vi "Editor Initialize.vi"(0 "Color Ramp Cluster in":T1={"Color Ramp Style"=enum."None", "Color Ramp Array"=[16711934, 393471, 57855, 4390754, 16449346, 16744722, 16711680], "Color Ramp Index"=[45, 91, 133, 175, 219, 255], "Interpolate?"=FALSE, "Logarithm?"=FALSE}, 1 "Fixed Slider Ref":refnum<vi>, 2 "Fixed Color Ref Array":refnum<vi>[](array[refnum]), 3 "Fixed Numeric Ref Array":refnum<vi>[](array[refnum]), 9 "Range In":cluster{"Max":sgl, "Min":sgl}, 11 "error in (no error)":errorcluster, 12 "Slider Ref Array":refnum<vi>[](array[refnum]), 13 "Color Ref Array":refnum<vi>[](array[refnum]), 14 "Numeric Ref Array":refnum<vi>[](array[refnum])) -> (4 "Color Ramp Cluster out":T1={"Color Ramp Style"=enum."None", "Color Ramp Array"=[16711934, 393471, 57855, 4390754, 16449346, 16744722, 16711680], "Color Ramp Index"=[45, 91, 133, 175, 219, 255], "Interpolate?"=FALSE, "Logarithm?"=FALSE}, 10 "Active Slider ID":i32, 15 "error out":errorcluster)   [LabVIEW 2020, in "3D Plot.lvclass"]
uses:
  3D Plot.lvclass
  Color Ramp Cluster.ctl
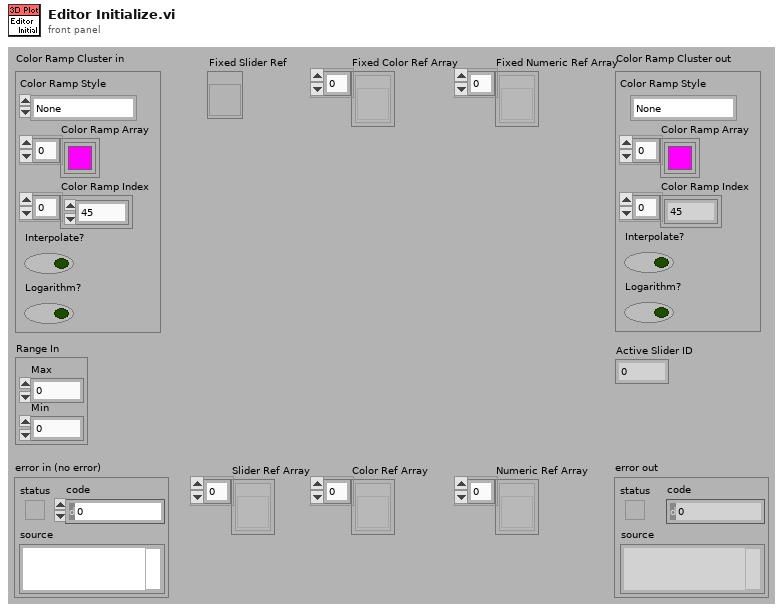
[diagram p1: front panel]
types:
  T1 = typedef "3D Plot.lvclass/Color Ramp Cluster.ctl" = cluster{"Color Ramp Style":enum16{"None", "Shaded", "Color spectrum", "Grey scale", "Custom"}, "Color Ramp Array":u32[], "Color Ramp Index":i32[], "Interpolate?":bool, "Logarithm?":bool}
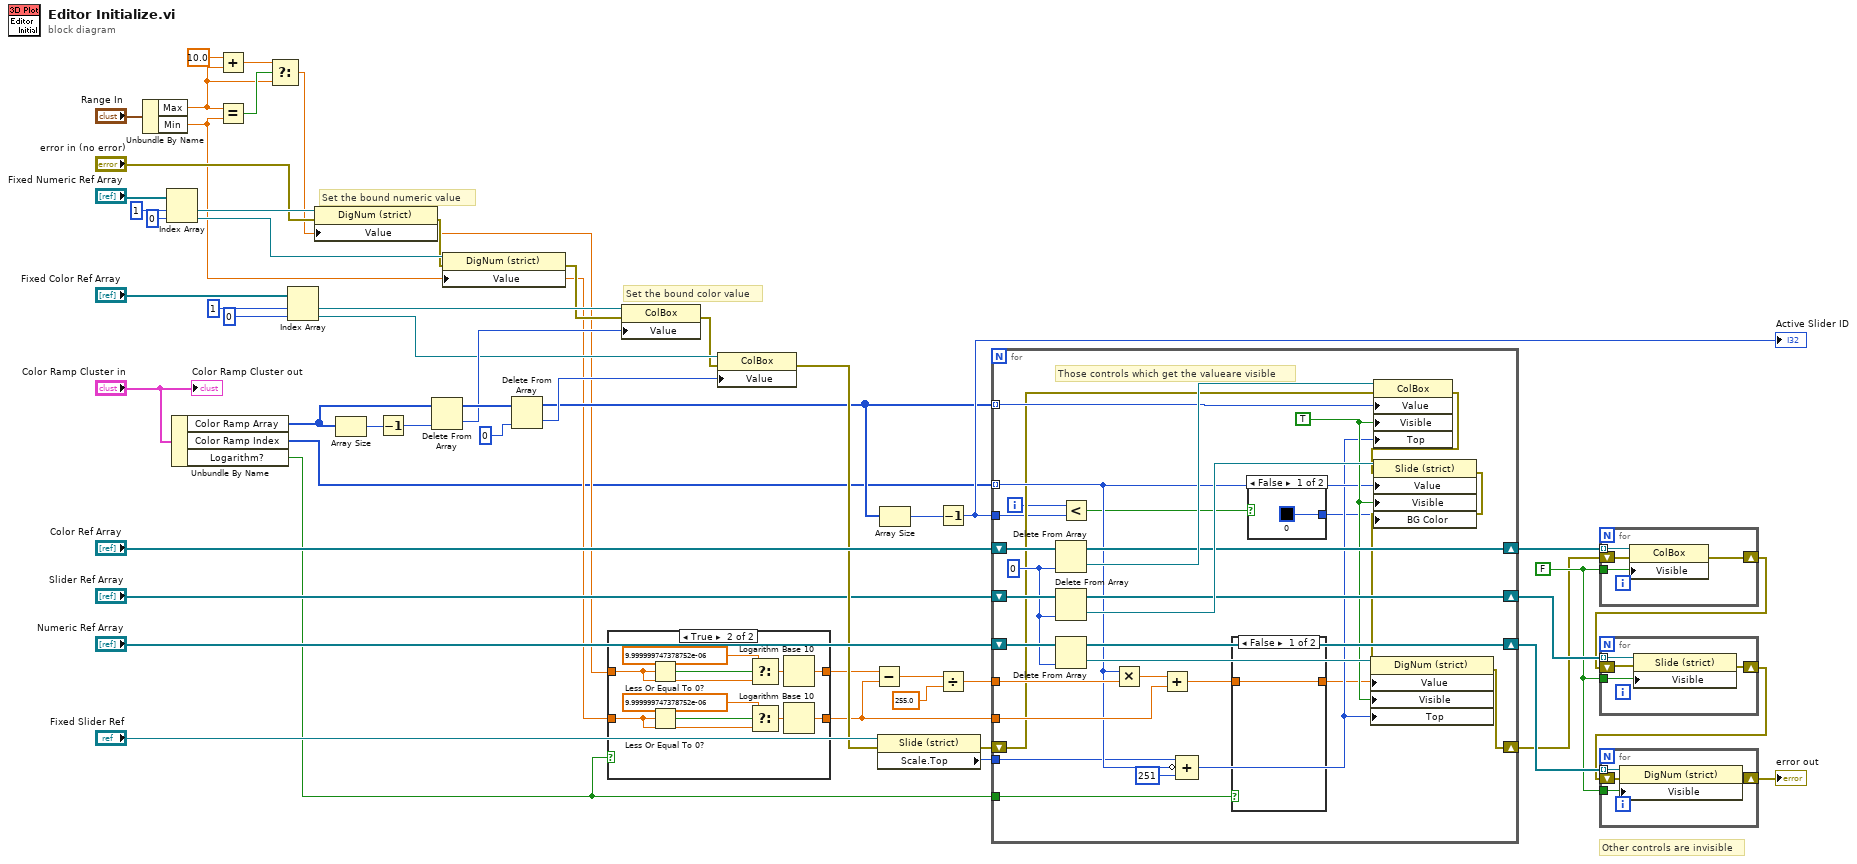
[diagram p0: block diagram]
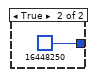
[diagram p3: hidden frame]
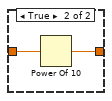
[diagram p4: hidden frame]
diagram:
  w30 = FALSE ("Visible")
  # "Other controls are invisible"
  # "Set the bound color value"
  # "Set the bound numeric value"
  n1 = Unbundle By Name("Range In") -> ("Max"=w6:sgl, "Min"=w10:sgl)
  n2 = Index Array(array="Fixed Numeric Ref Array", index #1=1 ("index"), index #2=0 ("index")) -> (element #1=w38:refnum<vi>, element #2=w37:refnum<vi>)
  n3 = Unbundle By Name("Color Ramp Cluster in") -> ("Color Ramp Array"=w3:u32[], "Color Ramp Index"=w2:i32[], "Logarithm?"=w1:bool)
  n4 = Add(x=sgl 10.0 ("t"), y=w6) -> (x+y=w5:sgl)
  n5 = Equal?(x=w6, y=w10) -> (x = y?=w9:bool)
  n6 = Select(t=w5, s=w9, f=w6) -> (s? t:f=w8:sgl)
  n7 = Index Array(array="Fixed Color Ref Array", index #1=1 ("index"), index #2=0 ("index")) -> (element #1=w45:refnum<vi>, element #2=w42:refnum<vi>)
  n8 = property class="DigNum (strict)"(reference=w38, error in="error in (no error)", "Value"=w8) -> (error out=w26:errorcluster)  [unwired: 1 out]
  n9 = Array Size(array=w3) -> (size(s)=w54:i32)
  n10 = Decrement(x=w54) -> (x-1=w52:i32)
  n11 = Delete From Array(array=w3, index=w52) -> (deleted portion=w51:u32, array with subset deleted=w53:u32[])  [unwired: 1 in]
  n12 = property class="DigNum (strict)"(reference=w37, error in=w26, "Value"=w10) -> (error out=w25:errorcluster)  [unwired: 1 out]
  n13 = Delete From Array(array=w53, index=0) -> (deleted portion=w49:u32, array with subset deleted=w12:u32[])  [unwired: 1 in]
  n14 = case shown="True" w1 {
    tunnel: w8 -> [w56 w57]
    tunnel: [w56 w66] -> w16
    tunnel: w10 -> [w55 w58]
    tunnel: [w55 w65] -> w15
    frame False {
    }
    frame True {
      n15 = Less Or Equal To 0?(x=w57) -> (x <= 0?=w61:bool)
      n16 = Less Or Equal To 0?(x=w58) -> (x <= 0?=w64:bool)
      n17 = Select(t=sgl 1e-05, s=w61, f=w57) -> (s? t:f=w60:sgl)
      n18 = Select(t=sgl 1e-05, s=w64, f=w58) -> (s? t:f=w59:sgl)
      n19 = Logarithm Base 10(1:w60) -> (0:w66:sgl)
      n20 = Logarithm Base 10(1:w59) -> (0:w65:sgl)
    }
  }
  n21 = property class="ColBox"(reference=w45, error in=w25, "Value"=w51) -> (error out=w24:errorcluster)  [unwired: 1 out]
  n22 = property class="ColBox"(reference=w42, error in=w24, "Value"=w49) -> (error out=w23:errorcluster)  [unwired: 1 out]
  n23 = Subtract(x=w16, y=w15) -> (x-y=w36:sgl)
  n24 = property class="Slide (strict)"(reference="Fixed Slider Ref", error in=w23) -> (error out=w22:errorcluster, "Scale.Top"=w29:i32)  [unwired: 1 out]
  n25 = Array Size(array=w12) -> (size(s)=w14:i32)
  n26 = Decrement(x=w14) -> (x-1=w13:i32)
  "Active Slider ID" <- w13
  n27 = Divide(x=w36, y=sgl 255.0) -> (x/y=w34:sgl)
  n28 = for {
    tunnel: w12 -> [w89] mode=indexing
    tunnel: w2 -> [w80] mode=indexing
    shift-right: [w84] -> w31
    shift-left: "Slider Ref Array" -> [w96]
    shift-right: [w83] -> w33
    shift-left: "Color Ref Array" -> [w94]
    shift-right: [w85] -> w32
    shift-left: "Numeric Ref Array" -> [w95]
    tunnel: w34 -> [w87]
    tunnel: w15 -> [w86]
    tunnel: w29 -> [w78]
    shift-right: [w74] -> w21
    shift-left: w22 -> [w77]
    tunnel: w1 -> [w71]
    tunnel: w13 -> [w68]
    i -> [w69]
    w82 = TRUE ("Visible")
    w90 = 0 ("index")
    # "Those controls which get the valueare visible"
    n29 = Delete From Array(array=w94, index=w90) -> (deleted portion=w92:refnum<vi>, array with subset deleted=w83:refnum<vi>[])  [unwired: 1 in]
    n30 = Delete From Array(array=w96, index=w90) -> (deleted portion=w93:refnum<vi>, array with subset deleted=w84:refnum<vi>[])  [unwired: 1 in]
    n31 = Delete From Array(array=w95, index=w90) -> (deleted portion=w91:refnum<vi>, array with subset deleted=w85:refnum<vi>[])  [unwired: 1 in]
    n32 = Less?(x=w69, y=w68) -> (x < y?=w67:bool)
    n33 = Multiply(x=w80, y=w87) -> (x*y=w88:sgl)
    n34 = Add(x=w88, y=w86) -> (x+y=w73:sgl)
    n35 = Compound Arithmetic op=ADD(w78, invert w80, 251 ("value")) -> (w79:i32)
    n36 = case shown="False" w71 {
      tunnel: w73 -> [w99 w101]
      tunnel: [w99 w100] -> w72
      frame False {
      }
      frame True {
        n37 = Power Of 10(x=w101) -> (10^x=w100:sgl)
      }
    }
    n38 = case shown="False" w67 {
      tunnel: [u32 0 u32 16448250] -> w70
      frame False {
      }
      frame True {
      }
    }
    n39 = property class="ColBox"(reference=w92, error in=w77, "Value"=w89, "Visible"=w82, "Top"=w79) -> (error out=w76:errorcluster)  [unwired: 1 out]
    n40 = property class="Slide (strict)"(reference=w93, error in=w76, "Value"=w80, "Visible"=w82, "BG Color"=w70) -> (error out=w75:errorcluster)  [unwired: 1 out]
    n41 = property class="DigNum (strict)"(reference=w91, error in=w75, "Value"=w72, "Visible"=w82, "Top"=w79) -> (error out=w74:errorcluster)  [unwired: 1 out]
  }
  n42 = for {
    tunnel: w30 -> [w105]
    tunnel: w33 -> [w104] mode=indexing
    shift-right: [w102] -> w20
    shift-left: w21 -> [w103]
    n43 = property class="ColBox"(reference=w104, error in=w103, "Visible"=w105) -> (error out=w102:errorcluster)  [unwired: 1 out]
  }
  n44 = for {
    tunnel: w30 -> [w109]
    tunnel: w31 -> [w108] mode=indexing
    shift-right: [w106] -> w19
    shift-left: w20 -> [w107]
    n45 = property class="Slide (strict)"(reference=w108, error in=w107, "Visible"=w109) -> (error out=w106:errorcluster)  [unwired: 1 out]
  }
  n46 = for {
    tunnel: w30 -> [w113]
    tunnel: w32 -> [w112] mode=indexing
    shift-right: [w110] -> w18
    shift-left: w19 -> [w111]
    n47 = property class="DigNum (strict)"(reference=w112, error in=w111, "Visible"=w113) -> (error out=w110:errorcluster)  [unwired: 1 out]
  }
  "error out" <- w18
  "Color Ramp Cluster out" <- "Color Ramp Cluster in"
